vi "createFileSubVI.vi"(0 "File Name":string caption="Beginning Text", 1 "File Comments":string, 4 "Path For File,\nManually Type the path, unless the file already exists.":path) -> (2 "refnum out":refnum<file>, 3 "File Path":path)   [LabVIEW 2012]
panel:
  out "error out":errorcluster
  out "error out 2":errorcluster
  in  "error in (no error)":errorcluster
  in  "error in":errorcluster
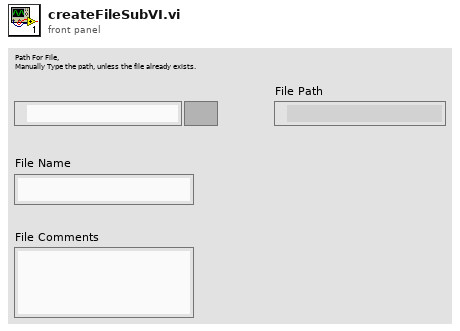
[diagram p1: front panel]
types:
  T1 = enum16{"open", "replace", "create", "open or create", "replace or create", "replace or create with confirmation"}
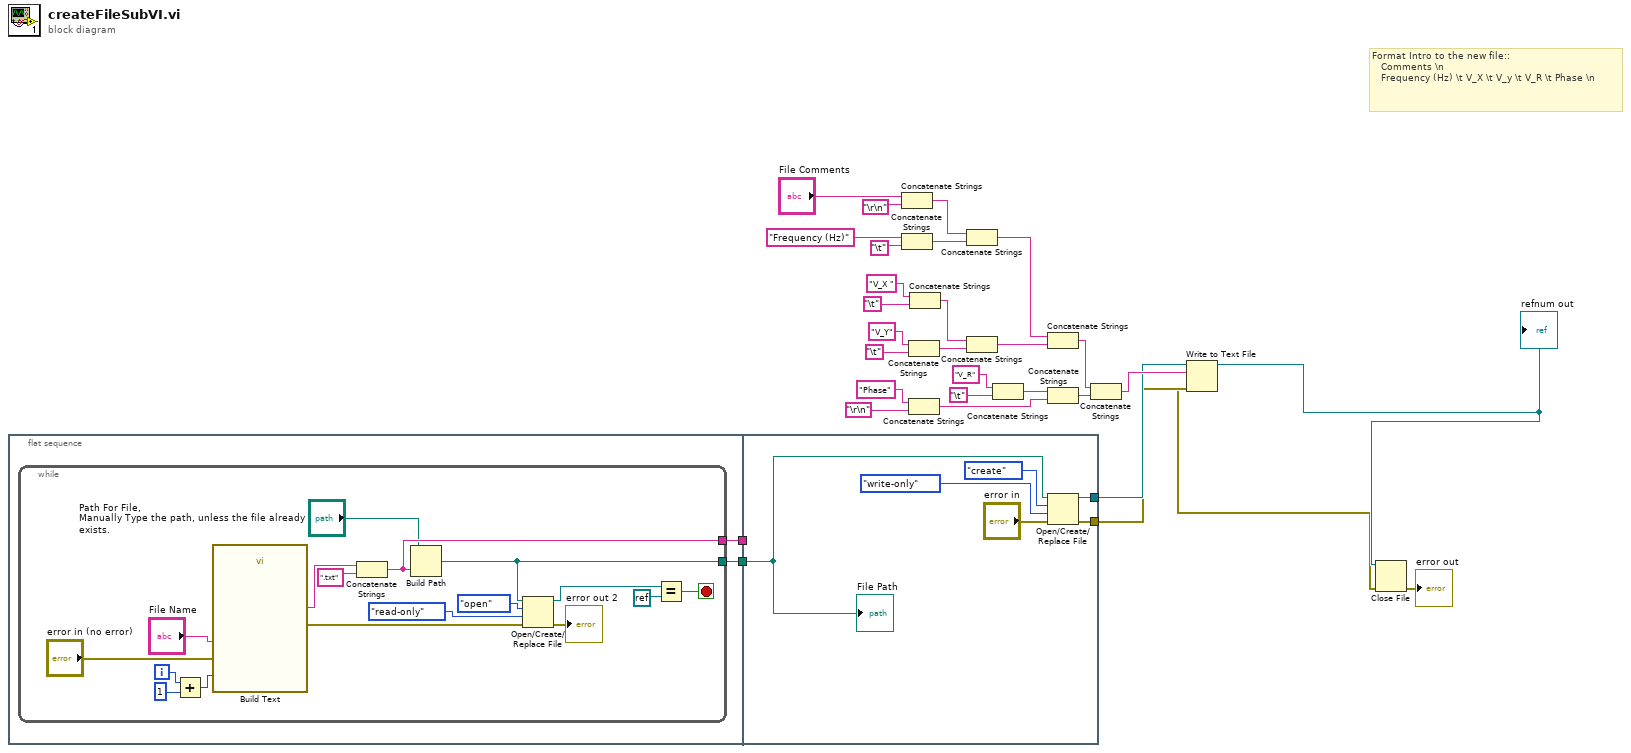
[diagram p0: block diagram]
diagram:
  # "Format Intro to the new file::\n   Comments \\n\n   Frequency (Hz) \\t V_X \\t V_y \\t V_R \\t Phase \\n"
  n1 = flat-sequence {
    tunnel: [w32] -> w7
    tunnel: [w31] -> w4
    tunnel: w7 -> [_]
    tunnel: [w55] -> w6
    tunnel: [w54] -> w5
    tunnel: w4 -> [w50]
    frame #0 {
      n2 = while {
        tunnel: [w35] -> w32
        tunnel: [w34] -> w31
        i -> [w45]
        stop <- w36 stop-if-true
        n3 = Add(x=w45, y=1) -> (x+y=w43:i32)
        n4 = call "Build Text"("Beginning Text"="File Name", "num"=w43, "error in (no error)"="error in (no error)") -> ("Result"=w49:string, "error out"=w40:errorcluster)  [unwired: 11 in]
        n5 = Concatenate Strings(w49, ".txt" ("string")) -> (w35:string)
        n6 = Build Path(base path="Path For File,\nManually Type the path, unless the file already exists.", name or relative path=w35) -> (appended path=w34:path)
        n7 = Open/Create/Replace File(file path (use dialog)=w34, error in=w40, operation (0:open)=T1."open", access (0:read/write)=enum16{"read/write", "read-only", "write-only"}."read-only") -> (refnum out=w38:refnum<file>, error out=→"error out 2":errorcluster)  [unwired: 2 in, 1 out]
        n8 = Equal?(x=w38, y=refnum<k0> refnum) -> (x = y?=w36:bool)
      }
    }
    frame #1 {
      n9 = Open/Create/Replace File(file path (use dialog)=w50, error in="error in", operation (0:open)=T1."create", access (0:read/write)=enum16{"read/write", "read-only", "write-only"}."write-only") -> (refnum out=w55:refnum<file>, error out=w54:errorcluster)  [unwired: 2 in, 1 out]
      "File Path" <- w50
    }
  }
  n10 = Concatenate Strings("File Comments", "\r\n") -> (w18:string)
  n11 = Concatenate Strings("Frequency (Hz)" ("string"), "\t") -> (w17:string)
  n12 = Concatenate Strings("V_Y" ("string"), "\t") -> (w15:string)
  n13 = Concatenate Strings("Phase" ("string"), "\r\n") -> (w13:string)
  n14 = Concatenate Strings("V_X " ("string"), "\t") -> (w16:string)
  n15 = Concatenate Strings(w18, w17) -> (w12:string)
  n16 = Concatenate Strings(w16, w15) -> (w11:string)
  n17 = Concatenate Strings("V_R" ("string"), "\t") -> (w14:string)
  n18 = Concatenate Strings(w12, w11) -> (w10:string)
  n19 = Concatenate Strings(w14, w13) -> (w9:string)
  n20 = Concatenate Strings(w10, w9) -> (w8:string)
  n21 = Write to Text File(file (use dialog)=w6, text=w8, error in=w5) -> (refnum out=w3:refnum<file>, error out=w2:errorcluster)  [unwired: 1 in, 1 out]
  "refnum out" <- w3
  n22 = Close File(refnum=w3, error in=w2) -> (error out=→"error out":errorcluster)  [unwired: 1 out]
